vi "Generate Sine Wave for Digital Audio.vi"(9 "phase":dbl, 10 "gain":dbl=0.5, 11 "frequency":dbl=0.5) -> (3 "Signal Properties":T1)   [LabVIEW 2023]
uses:
  <vilib>/PDM Acquisition Toolkit/host/Classes/Tasks/I2S Output/Control/SignalProperties.ctl
  <vilib>/PDM Acquisition Toolkit/host/Classes/Channels/I2S Ouput/Controls/GenerationChannelProperties.ctl
  <vilib>/Analysis/NI_AALBase.lvlib
  <vilib>/PDM Acquisition Toolkit/host/Classes/Channels/I2S Ouput/I2S Output Channel.lvclass
  <vilib>/PDM Acquisition Toolkit/host/Classes/Tasks/I2S Output/I2S Output Task.lvclass
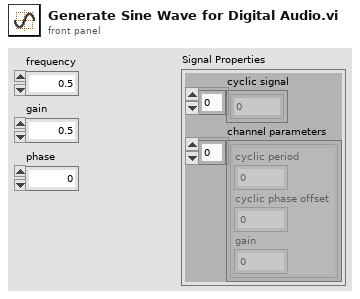
[diagram p1: front panel]
types:
  T1 = typedef "PDM Acquisition Class Library.lvlib/I2S Output Task.lvclass/SignalProperties.ctl" = cluster{"cyclic signal":dbl[], "channel parameters":T2[]}
  T2 = typedef "PDM Acquisition Class Library.lvlib/I2S Output Channel.lvclass/GenerationChannelProperties.ctl" = cluster{"cyclic period":dbl, "cyclic phase offset":dbl, "gain":dbl}
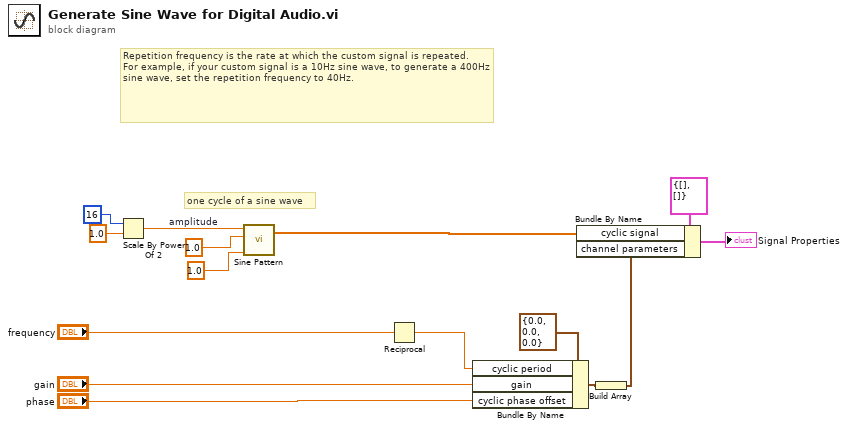
[diagram p0: block diagram]
diagram:
  w15 = 1.0  # amplitude
  # "one cycle of a sine wave"
  # "Repetition frequency is the rate at which the custom signal is repeated.\nFor example, if your custom signal is a 10Hz sine wave, to generate a 400Hz sine wave, set the repetition frequency to 40Hz."
  n1 = Scale By Power Of 2(n=i16 16, x=1.0) -> (x*2^n=w5:dbl)
  n2 = call <vilib>:"Sine Pattern.vi"("cycles"=1.0, "amplitude"=w15, "samples"=w5) -> ("Sinusoidal Pattern"=w9:dbl[])  [unwired: 1 in, 1 out]
  n3 = Reciprocal(x="frequency") -> (1/x=w2:dbl)
  n4 = Bundle By Name(cluster=T2 {"cyclic period"=0.0, "cyclic phase offset"=0.0, "gain"=0.0}, "cyclic period"=w2, "gain"="gain", "cyclic phase offset"="phase") -> (w7:T2)
  n5 = Build Array(w7) -> (w6:T2[])
  n6 = Bundle By Name(cluster=T1 {"cyclic signal"=[], "channel parameters"=[]} ("Signal Properties"), "cyclic signal"=w9, "channel parameters"=w6) -> (→"Signal Properties":T1)
